vi "Set Event (Raw).vi"(8 "error in (no error)":errorcluster, 9 "Raw data":i8[](array[numeric]), 10 "Event name":string, 11 "Event in":refnum<class "Event.lvclass">) -> (0 "error out":errorcluster, 3 "Event out":refnum<class "Event.lvclass">)   [LabVIEW 2010, in "MDSplus.lvlib" / "Event.lvclass"]
doc: "Issues an event passing a simple buffer of bytes (no Data)."
uses:
  <vilib>/MDSplus/Classes/Event_Class/Event.lvclass
  <vilib>/MDSplus/MDSobjectsLVShr.dll
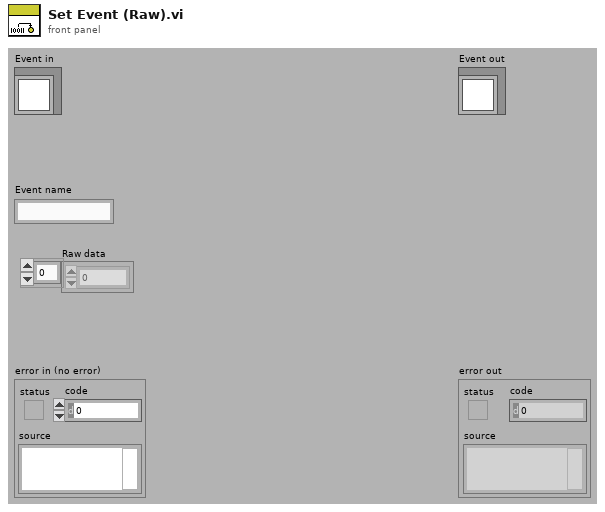
[diagram p1: front panel]
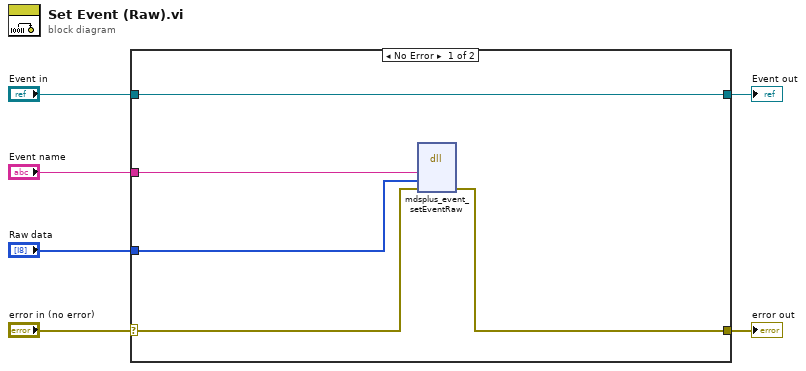
[diagram p0: block diagram]
diagram:
  n1 = case shown="No Error" "error in (no error)" {
    selector: "error in (no error)" -> [w10 w12]
    tunnel: [w9 w12] -> w5
    tunnel: [w8 w13] -> w4
    tunnel: "Event in" -> [w8 w13]
    tunnel: "Event name" -> [w11 _]
    tunnel: "Raw data" -> [w7 _]
    frame No Error {
      n2 = dll-call lib="C:/Program Files/National Instruments/LabVIEW 2010/vi.lib/MDSplus/MDSobjectsLVShr**.*" fn="mdsplus_event_setEventRaw"("evNameIn"=w11, "lvByteArrHdlIn"=w7, "error"=w10) -> ("error"=w9:errorcluster)  [unwired: 6 in, 2 out]
    }
    frame Error {
    }
  }
  "error out" <- w5
  "Event out" <- w4
